vi "LiftImmediate.vi"(7 "Description":string, 8 "Command Info In":T2, 9 "LiftArmCmd":dbl, 10 "LiftCmd":dbl, 11 "Operation":T1) -> (0 "Command Info Out":T2)   [LabVIEW 2017]
doc: "This template is useful for immediate subsystem actions that do not need deadband filtering\n\nBe sure to right-click and select New from Template and save with a new command name."
uses:
  <vilib>/Rock Robotics/WPI/Framework/Command Status Info.ctl
  <vilib>/Rock Robotics/WPI/Framework/Completion Status.ctl
  <vilib>/Rock Robotics/WPI/Framework/Completion Notifier.ctl
  Implementation/Lift Operations.ctl
  Implementation/Lift Setpoints.ctl
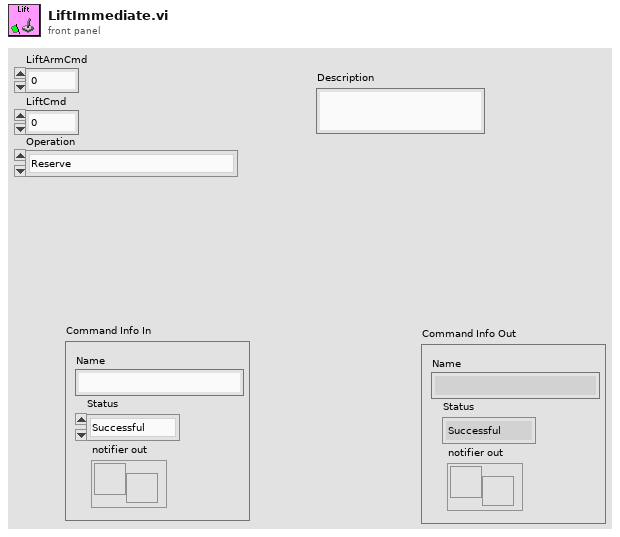
[diagram p1: front panel]
types:
  T1 = typedef "Lift Operations.ctl" = enum16{"Reserve", "Read Current", "Immediate"}
  T2 = typedef "Command Status Info.ctl" = cluster{"Name":string, "Status":T3, "notifier out":T4}
  T3 = typedef "Completion Status.ctl" = enum16{"Successful", "Aborted", "Incomplete"}
  T4 = typedef "Completion Notifier.ctl" = refnum<notifier>
  T5 = typedef "Lift Setpoints.ctl" = cluster{"Operation":T1, "LiftCmd":dbl, "LiftArmCmd":dbl}
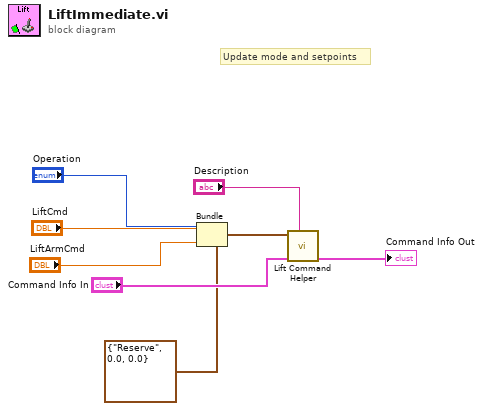
[diagram p0: block diagram]
diagram:
  # "Update mode and setpoints"
  n1 = Bundle(cluster=T5 {"Operation"=enum."Reserve", "LiftCmd"=0.0, "LiftArmCmd"=0.0} ("SubSystem Data"), "Operation"="Operation", "LiftCmd"="LiftCmd", "LiftArmCmd"="LiftArmCmd") -> (w4:T5)
  n2 = call "Lift Command Helper.vi"("Description"="Description", "Command Info In"="Command Info In", "SubSystem Data"=w4) -> ("Command Info Out"=→"Command Info Out":T2)  [unwired: 6 in, 2 out]
